vi "AVTCP-TCP Options FGV.vi"(4 "Value in":T1, 5 "Action":T2=enum."Read") -> (0 "Value out":T1, 1 "not empty":bool)   [LabVIEW 2020]
uses:
  AVTCP-FGV Action.ctl
  AVTCP-TCP Options.ctl
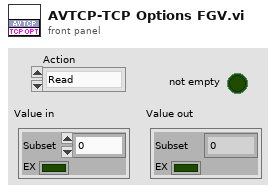
[diagram p1: front panel]
types:
  T1 = typedef "AVTCP-TCP Options.ctl" = cluster{"Subset":i32, "EX":bool}
  T2 = typedef "AVTCP-FGV Action.ctl" = enum16{"Init", "Write", "Read"}
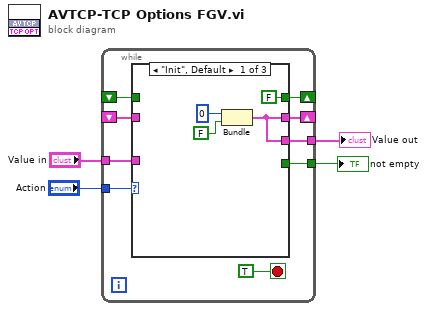
[diagram p0: block diagram]
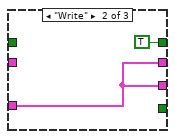
[diagram p2: hidden frame]
diagram:
  n1 = while {
    tunnel: "Action" -> [w13]
    tunnel: "Value in" -> [w11]
    shift-right: [w12] -> _
    shift-left: _ -> [w10]
    tunnel: [w9] -> w2
    shift-right: [w7] -> _
    shift-left: _ -> [w6]
    tunnel: [w5] -> w1
    stop <- TRUE stop-if-true
    n2 = case shown="\"Init\", Default" w13 {
      tunnel: [w17 w19 w21] -> w12
      tunnel: w11 -> [_ w19 _]
      tunnel: w10 -> [_ _ w21]
      tunnel: [w17 w19 w21] -> w9
      tunnel: [FALSE TRUE w20] -> w7
      tunnel: w6 -> [_ _ w20]
      tunnel: [_ _ w20] -> w5
      frame "Init", Default {
        n3 = Bundle(0, FALSE) -> (w17:cluster{i32, bool})  [unwired: 1 in]
      }
      frame "Write" {
      }
      frame "Read" {
      }
    }
  }
  "Value out" <- w2
  "not empty" <- w1
